vi "Core Actor - DISPLAY - Message (String).vi"(8 "error in (no error)":errorcluster, 9 "Value":string, 11 "Child_5_Class in":refnum<class "Error_Emgime_Class.lvclass">) -> (0 "error out":errorcluster, 3 "Child_5_Class out":refnum<class "Error_Emgime_Class.lvclass">)   [LabVIEW 2023, in "Error_Engine_Actor.lvlib" / "Error_Emgime_Class.lvclass"]
uses:
  Error_Emgime_Class.lvclass
  Abstraction_Interface_Class/Abstraction_Interface_Class.lvclass
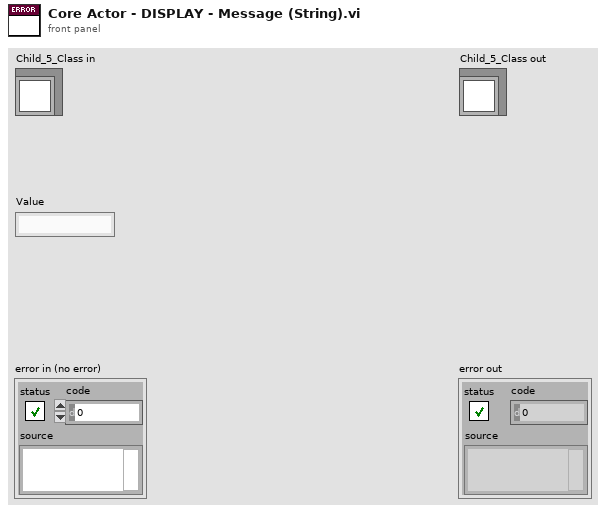
[diagram p1: front panel]
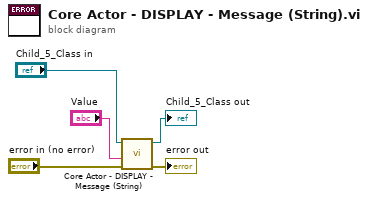
[diagram p0: block diagram]
diagram:
  n1 = call-parent "Core Actor - DISPLAY - Message (String).vi"("error in (no error)"="error in (no error)", "Value"="Value", "Interface_Class in"="Child_5_Class in") -> ("error out"=→"error out":errorcluster, "Interface_Class out"=→"Child_5_Class out":refnum<class "Error_Emgime_Class.lvclass">)  [unwired: 7 in]
